vi "get configured sequences.vi"(8 "error in (no error)":errorcluster, 11 "Simple Sequencer API in":refnum<class "Simple Sequencer API.lvclass">) -> (0 "error out":errorcluster, 2 "sequence definitions":T1[](array[typedef]), 3 "Simple Sequencer API out":refnum<class "Simple Sequencer API.lvclass">)   [LabVIEW 2014, in "Simple Sequencer API.lvclass"]
uses:
  Simple Sequencer API.lvclass
  module/configuration/sequence definition.ctl
  sequencer parent classes/action configuration parent/action configuration.lvclass
  Simple Sequencer API.lvclass/Simple Sequencer API.ctl
  module/configuration/Simple Sequencer TBM configuration.lvclass/Simple Sequencer TBM configuration.ctl
  module/configuration/Simple Sequencer TBM configuration.lvclass
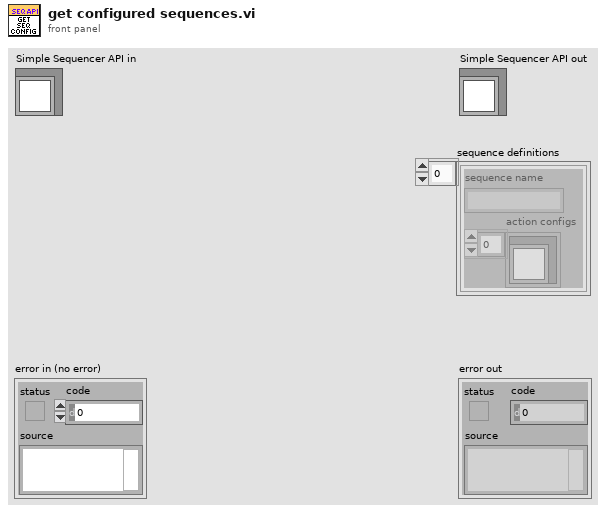
[diagram p1: front panel]
types:
  T1 = typedef "Simple Sequencer TBM configuration.lvclass/sequence definition.ctl" = cluster{"sequence name":string, "action configs":refnum<class "action configuration.lvclass">[]}
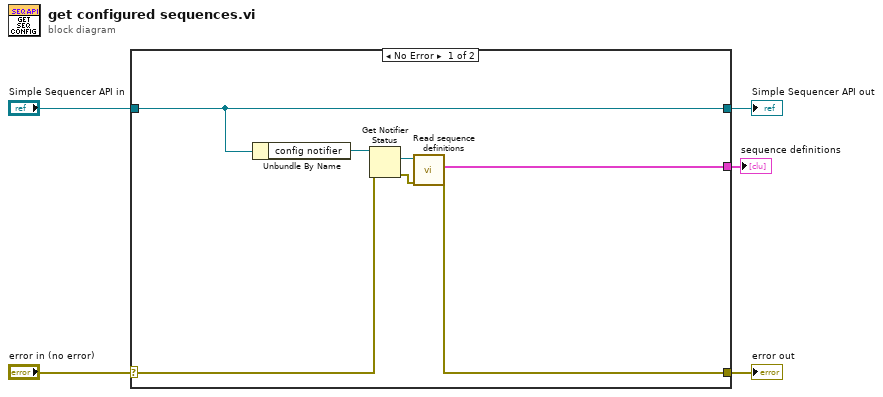
[diagram p0: block diagram]
diagram:
  n1 = case shown="No Error" "error in (no error)" {
    selector: "error in (no error)" -> [w10 w14]
    tunnel: [w6 w14] -> w4
    tunnel: [w11 w13] -> w2
    tunnel: "Simple Sequencer API in" -> [w11 w13]
    tunnel: [w8 _] -> w1
    frame No Error {
      n2 = Unbundle By Name(w11) -> ("config notifier"=w12:refnum<notifier>)
      n3 = Get Notifier Status(notifier=w12, error in (no error)=w10) -> (current notification=w9:refnum<class "Simple Sequencer TBM configuration.lvclass">, error out=w7:errorcluster)  [unwired: 3 out]
      n4 = call "Read sequence definitions.vi"("error in (no error)"=w7, "Simple Sequencer TBM configuration in"=w9) -> ("error out"=w6:errorcluster, "sequence definitions"=w8:T1[])  [unwired: 7 in, 1 out]
    }
    frame Error {
    }
  }
  "error out" <- w4
  "Simple Sequencer API out" <- w2
  "sequence definitions" <- w1
